vi "RecorderMainNoLoop.vi"(0 "NXT":T1={"Hardware"="NXT", "Flattened String"=""}, 1 "Close File? (False)":bool) -> (2 "NXT":T1={"Hardware"="NXT", "Flattened String"=""})   [LabVIEW 2010, in "Packet Recorder.lvlib"]
uses:
  Packet Recorder.lvlib
  <vilib>/NXT/Subs/LVHSConnector.ctl
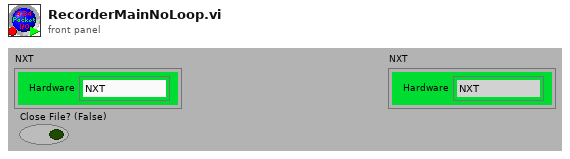
[diagram p1: front panel]
types:
  T1 = typedef "LVHSConnector.ctl" = cluster{"Hardware":string, "Flattened String":string}
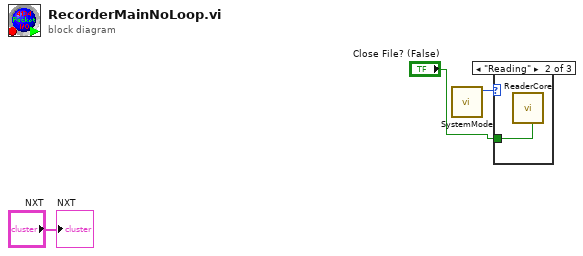
[diagram p0: block diagram]
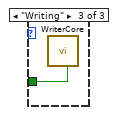
[diagram p3: hidden frame]
diagram:
  n1 = call "SystemMode.vi"() -> ("Mode"=w3:enum16{"Off", "Reading", "Writing"})  [unwired: 11 in]
  n2 = case shown="\"Reading\"" w3 {
    tunnel: "Close File? (False)" -> [_ w4 w5]
    frame "Off", Default {
    }
    frame "Reading" {
      n3 = call "ReaderCore.vi"("Close"=w4) -> ()  [unwired: 10 in, 1 out]
    }
    frame "Writing" {
      n4 = call "WriterCore.vi"("Close"=w5) -> ()  [unwired: 10 in, 1 out]
    }
  }
  "NXT" <- "NXT"
